vi "WindowArrayV1.00.vi"(0 "Searching center":dbl format="%.2f", 2 "X-axis":dbl[](array[numeric]) format="%.2f", 3 "The Data":dbl[](array[numeric]) format="%.2f", 5 "Window Width (point)":i32=80) -> (1 "scale":dbl format="%.2f", 4 "starting point":dbl format="%.2f", 6 "Closest peak position":dbl format="%.2f", 7 "X-Axis Subset":dbl[](array[numeric]) format="%.2f", 8 "Data Subset":dbl[](array[numeric]) format="%.2f")   [LabVIEW 2020]
doc: "Truncate the data around a peak. Normalize X-Axis so I can use the spline VI, and you can retrive the original X-Axis with *scale+StartingPoint."
uses:
  <vilib>/Analysis/NI_AALPro.lvlib
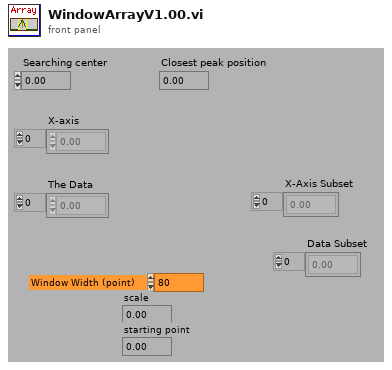
[diagram p1: front panel]
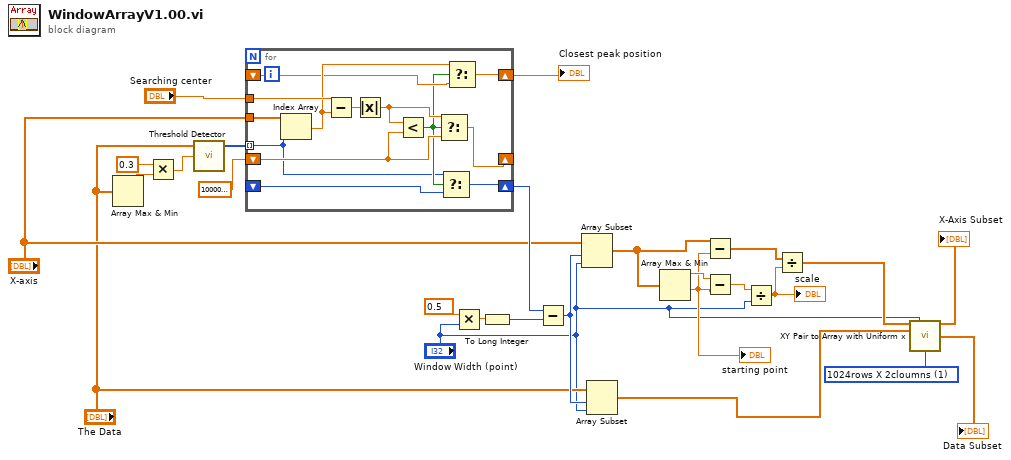
[diagram p0: block diagram]
diagram:
  w1 = u8 1 items=["No Change", "1024rows X 2cloumns", "1024X2 Fixed Endpoints"] ("Data Format")
  n1 = Array Max & Min(array="The Data") -> (max value=w21:dbl)  [unwired: 3 out]
  n2 = Multiply(x=0.3, y=w21) -> (x*y=w23:dbl)
  n3 = call <vilib>:"Threshold Detector.vi"("threshold"=w23, "X"="The Data") -> ("Indices"=w20:i32[])  [unwired: 1 in, 2 out]
  n4 = for {
    tunnel: w20 -> [w28] mode=indexing
    tunnel: "X-axis" -> [w39]
    tunnel: "Searching center" -> [w38]
    shift-right: [w34] -> _
    shift-left: 1000000000.0 ("x") -> [w35]
    shift-right: [w32] -> w26
    shift-left: _ -> [w31]
    shift-right: [w29] -> w19
    shift-left: _ -> [w27]
    n5 = Index Array(array=w39, index=w28) -> (element=w33:dbl)
    n6 = Subtract(x=w38, y=w33) -> (x-y=w37:dbl)
    n7 = Absolute Value(x=w37) -> (abs(x)=w36:dbl)
    n8 = Less?(x=w36, y=w35) -> (x < y?=w30:bool)
    n9 = Select(t=w36, s=w30, f=w35) -> (s? t:f=w34:dbl)
    n10 = Select(t=w28, s=w30, f=w27) -> (s? t:f=w29:i32)
    n11 = Select(t=w33, s=w30, f=w31) -> (s? t:f=w32:dbl)
  }
  "Closest peak position" <- w26
  n12 = Multiply(x=sgl 0.5 ("y"), y="Window Width (point)") -> (x*y=w18:sgl)
  n13 = To Long Integer(number=w18) -> (32bit integer=w17:i32)
  n14 = Subtract(x=w19, y=w17) -> (x-y=w14:i32)
  n15 = Array Subset(array="X-axis", index=w14, length="Window Width (point)") -> (w9:dbl[])
  n16 = Array Subset(array="The Data", index=w14, length="Window Width (point)") -> (w5:dbl[])
  n17 = Array Max & Min(array=w9) -> (max value=w12:dbl, min value=w10:dbl)  [unwired: 2 out]
  "starting point" <- w10
  n18 = Subtract(x=w9, y=w10) -> (x-y=w8:dbl[])
  n19 = Subtract(x=w12, y=w10) -> (x-y=w11:dbl)
  n20 = Divide(x=w11, y="Window Width (point)") -> (x/y=w7:dbl)
  "scale" <- w7
  n21 = Divide(x=w8, y=w7) -> (x/y=w6:dbl[])
  n22 = call "XY Pair to Array with Uniform x.vi"("x"=w6, "#Points"="Window Width (point)", "y"=w5, "Data Format"=w1) -> ("X output"=→"X-Axis Subset":dbl[], "Y output"=→"Data Subset":dbl[])  [unwired: 10 in]
